vi "Teleop.vi"(10 "Match Info":T1={"Autonomous Elapsed Seconds"=0.0, "TeleOp Elapsed Seconds"=0.0, "Disabled Elapsed Seconds"=0.0, "Visited Autonomous"=FALSE, "Visited TeleOp"=FALSE, "Visited Disabled"=FALSE, "Autonomous Settings"={"Autonomous Style"=enum."Independent", "VI Refnum"=refnum}}, 11 "Call Context":T2) -> ()   [LabVIEW 2016]
doc: "This VI is called for each TeleOp packet received from the DS where the robot is not disabled. It is often used to read from the joysticks and update I/O or to update setpoints for timed control loops. It should complete and return within 20 milliseconds or it may miss DS packets."
uses:
  <vilib>/Rock Robotics/WPI/DriverStation/WPI_DriverStationDerivedRobotMode.ctl
  <vilib>/Rock Robotics/WPI/DriverStation/WPI_DriverStationMatch Info.ctl
  <vilib>/Rock Robotics/WPI/Utilities/WPI_GetSetVariantRefNum.vi
  <vilib>/Rock Robotics/WPI/Ultrasonic/WPI_SonarMB1010DigitalRefNum Registry Get.vi
  <vilib>/Rock Robotics/WPI/Ultrasonic/WPI_SonarMB1010DigitalGetRange.vi
  FRC SimulatedRSC/Positions.vi
panel:
  out "Distance":dbl format="%#_13g"
  out "Gyro Angle":dbl format="%#_13g"
  in  "Set RPM":dbl=7000.0 format="%#_13g"
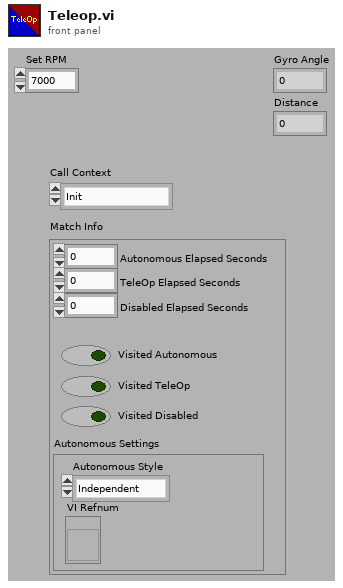
[diagram p1: front panel]
types:
  T1 = typedef "WPI_DriverStationMatch Info.ctl" = cluster{"Autonomous Elapsed Seconds":dbl, "TeleOp Elapsed Seconds":dbl, "Disabled Elapsed Seconds":dbl, "Visited Autonomous":bool, "Visited TeleOp":bool, "Visited Disabled":bool, "Autonomous Settings":cluster{"Autonomous Style":enum16{"Iterative", "Independent"}, "VI Refnum":refnum<vi>}}
  T2 = typedef "WPI_DriverStationDerivedRobotMode.ctl" = enum16{"Init", "Execute", "Stop"}
  T3 = typedef "WPI_JoystickDevRef.ctl" = cluster{"Device":T4}
  T4 = typedef "WPI_JoystickDeviceEnum.ctl" = enum16{"USB 0", "USB 1", "USB 2", "USB 3", "USB 4", "USB 5"}
  T5 = typedef "WPI_SonarMB1010DigitalDeviceRef.ctl" = cluster{"CounterDevRef":T6, "Scaling factor (s/in)":dbl}
  T6 = typedef "WPI_CounterDevRef.ctl" = cluster{"DevStatus":errorcluster, "CntIndex":T7}
  T7 = typedef "FPGA_CounterCtrSystemIndex.ctl" = enum8{"Ctr 0", "Ctr 1", "Ctr 2", "Ctr 3", "Ctr 4", "Ctr 5", "Ctr 6", "Ctr 7", "Invalid"}
  T8 = typedef "WPI_GyroDevRef.ctl" = cluster{"DevStatus":errorcluster, "Analog Channel":T9, "Offset":dbl, "Gain (VoltsPerDegree/Second)":dbl, "Gyro Type":enum16{"Analog", "XRS450"}, "Handle":i32, "SPI Bus":T10, "Device Found":bool, "Sample Rate":dbl, "Calibrate On Open":bool}
  T9 = typedef "FPGA_AIChannel.ctl" = enum8{"AI 0", "AI 1", "AI 2", "AI 3", "AI MXP 0", "AI MXP 1", "AI MXP 2", "AI MXP 3", "Invalid"}
  T10 = typedef "spi_bus.ctl" = enum16{"SPI On-Board, CS0", "SPI On-Board, CS1", "SPI On-Board, CS2", "SPI On-Board, CS3", "SPI MXP", "Invalid"}
  T11 = typedef "WPI_MotorControlDeviceRef.ctl" = cluster{"DeviceStatus":errorcluster, "Type":T12, "PWM":cluster{"PWM Channel":T13, "DeadBand":T14}, "CAN":cluster{"Device Number":u8, "SetOutput VI Ref":variant, "GetOutput VI Ref":variant, "Enable VI Ref":variant, "Disable VI Ref":variant, "Data":variant}, "Invert":bool}
  T12 = typedef "WPI_MotorControlType.ctl" = enum16{"PWM", "CAN"}
  T13 = typedef "FPGA_DIOPWMChannel.ctl" = enum8{"PWM 0", "PWM 1", "PWM 2", "PWM 3", "PWM 4", "PWM 5", "PWM 6", "PWM 7", "PWM 8", "PWM 9", "PWM MXP 0", "PWM MXP 1", "PWM MXP 2", "PWM MXP 3", "PWM MXP 4", "PWM MXP 5", "PWM MXP 6", "PWM MXP 7", "PWM MXP 8", "PWM MXP 9", "Invalid"}
  T14 = typedef "WPI_PWMDeadband.ctl" = cluster{"Name":string, "maxPositivePwm":i32, "minPositivePwm":i32, "centerPwm":i32, "maxNegativePwm":i32, "minNegativePwm":i32, "angularRange":u16}
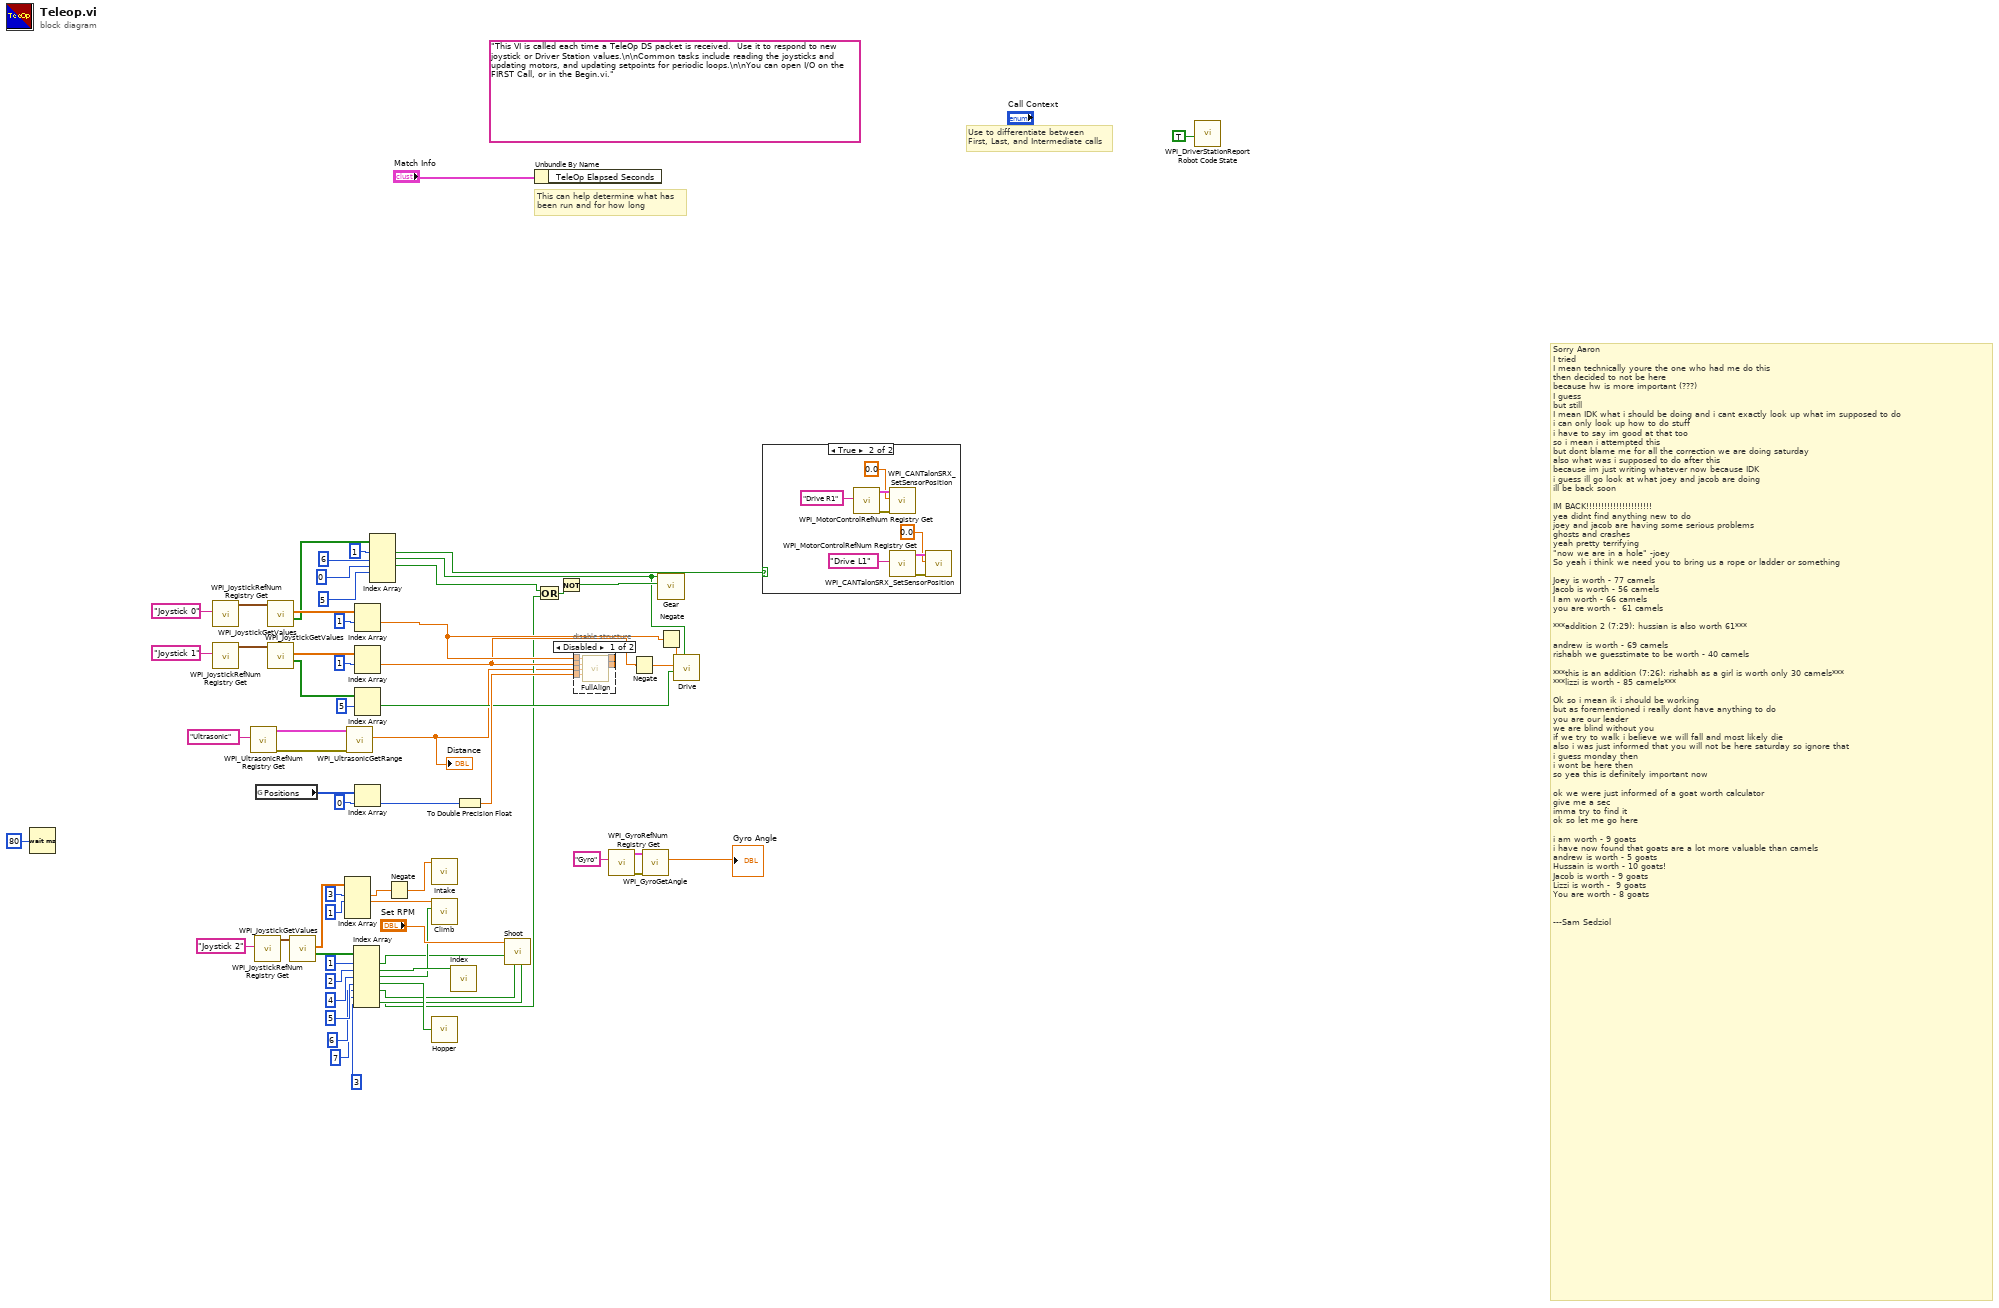
[diagram p0: block diagram]
diagram:
  (unwired) "This VI is called each time a TeleOp DS packet is received.  Use it to respond to new joystick or Driver Station values.\n\nCommon tasks include reading the joysticks and updating motors, and updating setpoints for periodic loops.\n\nYou can open I/O on the FIRST Call, or in the Begin.vi."
  # "Sorry Aaron\nI tried\nI mean technically youre the one who had me do this\nthen decided to not be here\nbecause hw is more important (???)\nI guess\nbut still\nI mean IDK what i should be doing and i cant exactly look up what im supposed to do\ni can only look up how to do stuff\ni have to say im good at that too\nso i mean i attempted this\nbut dont blame me for all the correction we are doing saturday\nalso what was i supposed to do after this\nbecause im just writing whatever now because IDK\ni guess ill go look at what joey and jacob are doing\nill be back soon\n\nIM BACK!!!!!!!!!!!!!!!!!!!!!!\nyea didnt find anything new to do\njoey and jacob are having some serious problems\nghosts and crashes\nyeah pretty terrifying\n\"now we are in a hole\" -joey\nSo yeah i think we need you to bring us a rope or ladder or something\n\nJoey is worth - 77 camels\nJacob is worth - 56 camels\nI am worth - 66 camels\nyou are worth -  61 camels \n\n***addition 2 (7:29): hussian is also worth 61***\n\nandrew is worth - 69 camels\nrishabh we guesstimate to be worth - 40 camels\n\n***this is an addition (7:26): rishabh as a girl is worth only 30 camels***\n***lizzi is worth - 85 camels***\n\nOk so i mean ik i should be working\nbut as forementioned i really dont have anything to do\nyou are our leader\nwe are blind without you\nif we try to walk i believe we will fall and most likely die\nalso i was just informed that you will not be here saturday so ignore that\ni guess monday then\ni wont be here then\nso yea this is definitely important now\n\nok we were just informed of a goat worth calculator\ngive me a sec \nimma try to find it\nok so let me go here\n\ni am worth - 9 goats\ni have now found that goats are a lot more valuable than camels\nandrew is worth - 5 goats\nHussain is worth - 10 goats! \nJacob is worth - 9 goats\nLizzi is worth -  9 goats\nYou are worth - 8 goats\n\n\n---Sam Sedziol"
  # "Use to differentiate between\nFirst, Last, and Intermediate calls"
  # "This can help determine what has\nbeen run and for how long"
  n1 = Wait (ms)(milliseconds to wait=u32 80) -> ()  [unwired: 1 out]
  n2 = call <vilib>:"WPI_JoystickRefNum Registry Get.vi"("refnum name"="Joystick 0") -> ("JoystickDevRef"=w39:T3)  [unwired: 1 in, 9 out]
  n3 = call <vilib>:"WPI_JoystickRefNum Registry Get.vi"("refnum name"="Joystick 1") -> ("JoystickDevRef"=w38:T3)  [unwired: 1 in, 9 out]
  n4 = call-poly <vilib>:"WPI_UltrasonicRefNum Registry Get.vi"("refnum name"="Ultrasonic") -> ("error out"=w49:errorcluster, "SonarMB1010DigitalDevRef"=w50:T5)  [unwired: 9 in]
  n5 = call <vilib>:"WPI_JoystickRefNum Registry Get.vi"("refnum name"="Joystick 2") -> ("JoystickDevRef"=w58:T3)  [unwired: 1 in, 9 out]
  n6 = global read "Positions.vi" "Positions"() -> (w40:i32[])
  n7 = call <vilib>:"WPI_JoystickGetValues.vi"("JoystickDevRef"=w39) -> ("Buttons"=w54:bool[], "Axes"=w61:dbl[])  [unwired: 6 in, 3 out]
  n8 = call <vilib>:"WPI_JoystickGetValues.vi"("JoystickDevRef"=w38) -> ("Buttons"=w55:bool[], "Axes"=w60:dbl[])  [unwired: 6 in, 3 out]
  n9 = call <vilib>:"WPI_JoystickGetValues.vi"("JoystickDevRef"=w58) -> ("Buttons"=w56:bool[], "Axes"=w57:dbl[])  [unwired: 6 in, 3 out]
  n10 = Index Array(array=w57, index #1=3 ("index"), index #2=1 ("index")) -> (element #1=w51:dbl, element #2=w42:dbl)  [unwired: 2 in, 2 out]
  n11 = call-poly <vilib>:"WPI_UltrasonicGetRange.vi"("error in"=w49, "SonarMB1010DigitalDevRef"=w50) -> ("Distance"=w1:dbl)  [unwired: 7 in, 2 out]
  "Distance" <- w1
  n12 = Index Array(array=w56, index #1=1 ("index"), index #2=2 ("index"), index #3=4 ("index"), index #4=5 ("index"), index #5=6 ("index"), index #6=7 ("index"), index #7=3 ("index")) -> (element #1=w16:bool, element #2=w41:bool, element #3=w24:bool, element #4=w23:bool, element #5=w13:bool, element #6=w12:bool, element #7=w7:bool)
  n13 = Index Array(array=w61, index #1=1 ("index")) -> (element #1=w18:dbl)  [unwired: 1 in, 1 out]
  n14 = Index Array(array=w60, index #1=1 ("index")) -> (element #1=w17:dbl)  [unwired: 1 in, 1 out]
  n15 = Index Array(array=w55, index #1=5 ("index")) -> (element #1=w19:bool)  [unwired: 1 in, 1 out]
  n16 = Index Array(array=w40, index=0) -> (element=w44:i32)
  n17 = Index Array(array=w54, index #1=1 ("index"), index #2=6 ("index"), index #3=0 ("index"), index #4=5 ("index")) -> (element #1=w47:bool, element #2=w2:bool, element #3=w11:bool)  [unwired: 1 in, 2 out]
  n18 = Negate(x=w51) -> (-x=w33:dbl)
  n19 = call "Intake.vi"("Effort"=w33) -> ()  [unwired: 11 in]
  n20 = call "Climb.vi"("Backwards?"=w24, "Effort"=w42) -> ()  [unwired: 10 in]
  n21 = call "Hopper.vi"("Hopper?"=w23) -> ()  [unwired: 4 in]
  n22 = call "Index.vi"("Index?"=w41) -> ()  [unwired: 11 in]
  n23 = To Double Precision Float(number=w44) -> (double precision float=w43:dbl)
  n24 = call "Shoot.vi"("Icrement Up"=w12, "Icrement Down"=w13, "Override?"=w16, "Set RPM"="Set RPM") -> ()  [unwired: 8 in]
  n25 = Unbundle By Name("Match Info") -> ()  [unwired: 1 out]
  n26 = Or(x=w11, y=w7) -> (x .or. y?=w10:bool)
  n27 = Not(x=w10) -> (.not. x?=w9:bool)
  n28 = disable-structure shown="Disabled" {
    disable-tunnel: w18 -> [w70 _]
    disable-tunnel: w17 -> [w69 _]
    disable-tunnel: w1 -> [w68 _]
    disable-tunnel: w43 -> [w67 _]
    disable-tunnel: [w66 _] -> _
    disable-tunnel: [w65 _] -> _
    frame Disabled {
      n29 = call "FullAlign.vi"("Joystick 0"=w70, "Joystick 1"=w69, "Distance"=w68, "Angle"=w67) -> ("Right Motor"=w65:dbl, "Left Motor"=w66:dbl)  [unwired: 9 in, 1 out]
    }
    frame Enabled {
    }
  }
  n30 = call <vilib>:"WPI_GyroRefNum Registry Get.vi"("refnum name"="Gyro") -> ("error out"=w6:errorcluster, "GyroDevRef"=w5:T8)  [unwired: 9 in]
  n31 = Negate(x=w17) -> (-x=w29:dbl)
  n32 = call <vilib>:"WPI_GyroGetAngle.vi"("error in"=w6, "GyroDevRef"=w5) -> ("Angle"=→"Gyro Angle":dbl)  [unwired: 5 in, 4 out]
  n33 = call "Gear.vi"("Gear1?"=w9, "Gear0?"=w2) -> ()  [unwired: 10 in]
  n34 = Negate(x=w18) -> (-x=w30:dbl)
  n35 = call "Drive.vi"("Slow?"=w2, "SwitchDir"=w19, "Drive L"=w29, "Drive R"=w30) -> ()  [unwired: 8 in]
  n36 = case shown="True" w47 {
    frame False {
    }
    frame True {
      n37 = call <vilib>:"WPI_MotorControlRefNum Registry Get.vi"("refnum name"="Drive R1") -> ("error out"=w73:errorcluster, "MotorControlDevRef"=w72:T11)  [unwired: 9 in]
      n38 = call <vilib>:"WPI_CANTalonSRX_SetSensorPosition.vi"("error in (no error)"=w73, "New Sensor Position"=0.0, "CAN Talon SRX Ref"=w72) -> ()  [unwired: 7 in, 2 out]
      n39 = call <vilib>:"WPI_MotorControlRefNum Registry Get.vi"("refnum name"="Drive L1") -> ("error out"=w75:errorcluster, "MotorControlDevRef"=w76:T11)  [unwired: 9 in]
      n40 = call <vilib>:"WPI_CANTalonSRX_SetSensorPosition.vi"("error in (no error)"=w75, "New Sensor Position"=0.0, "CAN Talon SRX Ref"=w76) -> ()  [unwired: 7 in, 2 out]
    }
  }
  n41 = call <vilib>:"WPI_DriverStationReport Robot Code State.vi"("TeleOp"=TRUE ("Autonomous")) -> ()  [unwired: 10 in, 1 out]
